vi "4Pi Focus Lock - Values Organize Plot Data.vi"(0 "Target 01":dbl, 2 "Value Limit":dbl, 7 "Current 1":dbl, 9 "Current 2":dbl, 11 "Stage Position":dbl) -> (8 "output cluster":T1)   [LabVIEW 2021]
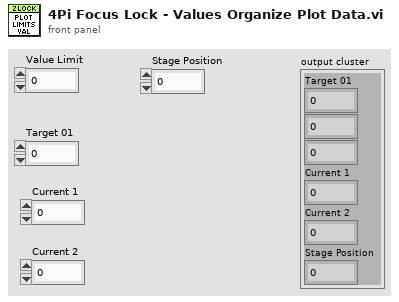
[diagram p1: front panel]
types:
  T1 = cluster{"Target 01":dbl, dbl, dbl, "Current 1":dbl, "Current 2":dbl, "Stage Position":dbl}
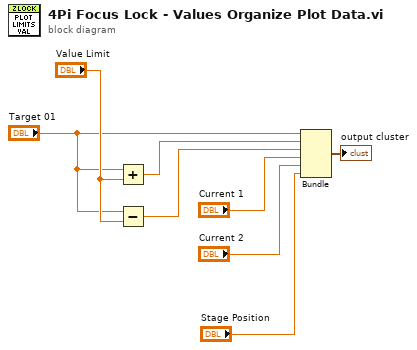
[diagram p0: block diagram]
diagram:
  n1 = Add(x="Target 01", y="Value Limit") -> (x+y=w6:dbl)
  n2 = Subtract(x="Target 01", y="Value Limit") -> (x-y=w5:dbl)
  n3 = Bundle("Target 01"="Target 01", w6, w5, "Current 1"="Current 1", "Current 2"="Current 2", "Stage Position"="Stage Position") -> (→"output cluster":T1)  [unwired: 1 in]
